vi "Write Listbox.vi"(5 "Action":T1, 7 "eHS Core Index":T2, 8 "Error In":errorcluster, 10 "Multicolumn Listbox Ref In":refnum<vi>, 11 "eHS Matrix Generation Session Ref In":refnum<data-value>) -> (0 "Error Out":errorcluster, 2 "Multicolumn Listbox Ref Out":refnum<vi>, 3 "eHS Matrix Generation Session Ref Out":refnum<data-value>)   [LabVIEW 2017]
uses:
  <vilib>/OPAL-RT/eHS Toolkit/eHS Matrix Generation/_Controls/eHS Core Index.ctl
  <vilib>/OPAL-RT/eHS Toolkit/eHS Matrix Generation/_Controls/eHS Matrix Generation Session.ctl
  <vilib>/OPAL-RT/eHS Toolkit/eHS Matrix Generation/_Controls/eHS Target Information.ctl
  <vilib>/OPAL-RT/eHS Toolkit/eHS Matrix Generation/_Controls/eHS Matrix Generation Parameters.ctl
  <vilib>/OPAL-RT/eHS Toolkit/eHS Matrix Generation/_Controls/eHS Circuit Analysis Data.ctl
  <vilib>/OPAL-RT/eHS Toolkit/eHS Matrix Generation/_Controls/eHS Core Settings.ctl
  <vilib>/OPAL-RT/eHS Toolkit/eHS Matrix Generation/_Controls/eHS Form Factor.ctl
  <vilib>/OPAL-RT/eHS Toolkit/eHS Matrix Generation/_Controls/eHS Model Information.ctl
  ListBox Action.ctl
  <vilib>/OPAL-RT/eHS Toolkit/eHS Matrix Generation/eHS Matrix Generation.lvlib
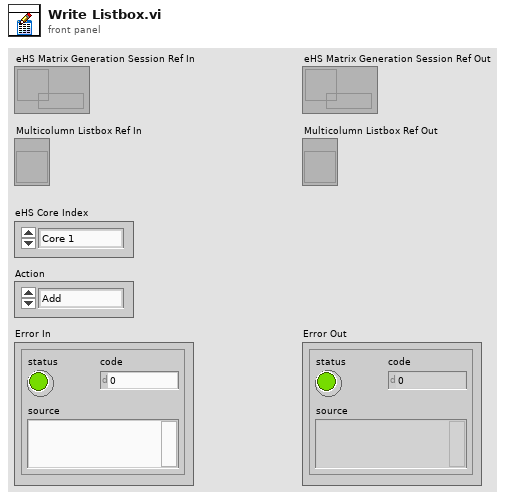
[diagram p1: front panel]
types:
  T1 = typedef "ListBox Action.ctl" = enum16{"Add", "Overwrite"}
  T2 = typedef "OPAL-RT eHS.lvlib/eHS Matrix Generation.lvlib/eHS Core Index.ctl" = enum16{"Core 1", "Core 2", "Core 3", "Core 4", "Core 5", "Core 6", "Core 7", "Core 8", "Core 9", "Core 10"}
  T3 = typedef "OPAL-RT eHS.lvlib/eHS Matrix Generation.lvlib/eHS Form Factor.ctl" = enum16{"eHSx16", "eHSx32", "eHSx64"}
  T4 = typedef "OPAL-RT eHS.lvlib/eHS Matrix Generation.lvlib/eHS Circuit Analysis Data.ctl" = cluster{"Number of Switches":string, "Desired Ts":string, "Gs":dbl[], "Min Ts":string}
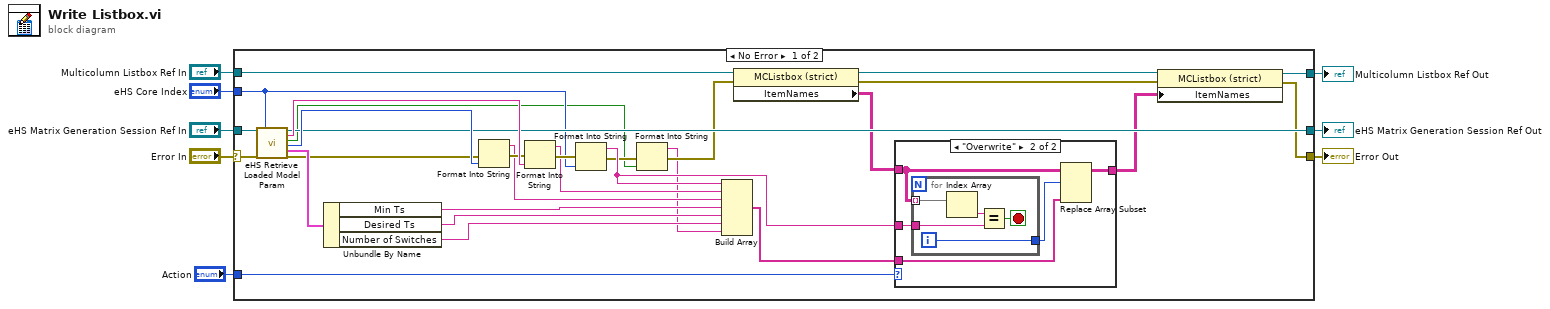
[diagram p0: block diagram]
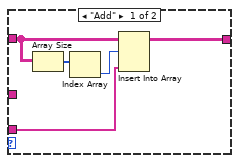
[diagram p2: hidden frame]
diagram:
  n1 = case shown="No Error" "Error In" {
    selector: "Error In" -> [w34 w55]
    tunnel: [w19 w55] -> w7
    tunnel: "Multicolumn Listbox Ref In" -> [w37 w54]
    tunnel: [w35 w54] -> w5
    tunnel: "eHS Core Index" -> [w16 _]
    tunnel: "eHS Matrix Generation Session Ref In" -> [w33 w53]
    tunnel: [w21 w53] -> w2
    tunnel: "Action" -> [w18 _]
    frame No Error {
      n2 = call <vilib>:"eHS Retrieve Loaded Model Param.vi"("eHS Matrix Generation Session Ref In"=w33, "Error In"=w34, "eHS Core Index"=w16) -> ("eHS Matrix Generation Session Ref Out"=w21:refnum<data-value>, "Model Name"=w30:string, "Support Scenarios"=w11:bool, "eHS Form Factor"=w28:T3, "eHS Circuit Analysis Data"=w26:T4, "Error Out"=w22:errorcluster)  [unwired: 10 in, 1 out]
      n3 = Unbundle By Name(w26) -> ("Min Ts"=w25:string, "Desired Ts"=w24:string, "Number of Switches"=w23:string)
      n4 = Format Into String(error in=w22, w28) -> (resulting string=w27:string, error out=w29:errorcluster)  [unwired: 2 in]
      n5 = Format Into String(error in=w29, w30) -> (resulting string=w31:string, error out=w32:errorcluster)  [unwired: 2 in]
      n6 = Format Into String(error in=w32, w16) -> (resulting string=w15:string, error out=w14:errorcluster)  [unwired: 2 in]
      n7 = Format Into String(error in=w14, w11) -> (resulting string=w12:string, error out=w13:errorcluster)  [unwired: 2 in]
      n8 = Build Array(w15, w31, w27, w25, w24, w23, w12) -> (w10:string[])
      n9 = property on="Property Node" class="MCListbox (strict)"(reference=w37, error in=w13) -> (reference out=w36:refnum<vi>, error out=w20:errorcluster, "ItemNames"=w17:string[][])
      n10 = case shown="\"Overwrite\"" w18 {
        tunnel: w17 -> [w41 w43]
        tunnel: w15 -> [_ w47]
        tunnel: w10 -> [w40 w44]
        tunnel: [w38 w46] -> w9
        frame "Add" {
          n11 = Array Size(array=w41) -> (size(s)=w42:i32[])
          n12 = Index Array(array=w42) -> (element=w39:i32)  [unwired: 1 in]
          n13 = Insert Into Array(array=w41, index (row)=w39, new element=w40) -> (w38:string[][])  [unwired: 1 in]
        }
        frame "Overwrite" {
          n14 = for {
            tunnel: w43 -> [w51] mode=indexing
            tunnel: w47 -> [w52]
            tunnel: [w48] -> w45
            i -> [w48]
            stop <- w49 stop-if-true
            n15 = Index Array(array=w51) -> (element=w50:string)  [unwired: 1 in]
            n16 = Equal?(x=w50, y=w52) -> (x = y?=w49:bool)
          }
          n17 = Replace Array Subset(array=w43, new element=w44, index (row)=w45) -> (w46:string[][])  [unwired: 1 in]
        }
      }
      n18 = property on="Property Node" class="MCListbox (strict)"(reference=w36, error in=w20, "ItemNames"=w9) -> (reference out=w35:refnum<vi>, error out=w19:errorcluster)
    }
    frame Error {
    }
  }
  "Multicolumn Listbox Ref Out" <- w5
  "Error Out" <- w7
  "eHS Matrix Generation Session Ref Out" <- w2
